vi "Configure Width Trigger Source [WT] Core.vi"(0 "IVI_Scope in":refnum<class "IVI_Scope.lvclass">, 1 "trigger source (\"CHANNEL1\")":string(combo)="CHANNEL1", 2 "trigger level (0.0 V)":dbl[unit] format="%.3f", 3 "width condition (Within)":i32(ring)=1 items=["Within"=1, "Outside"=2], 4 "width polarity (Positive)":i32(ring)=1 items=["Positive"=1, "Negative"=2], 5 "error in (no error)":errorcluster, 6 "width low threshold (1.0 E-9 V)":dbl[unit]=1e-09 format="%^.3e", 8 "width high threshold (2.0 E-9 V)":dbl[unit]=2e-09 format="%^.3e") -> (14 "IVI_Scope out":refnum<class "IVI_Scope.lvclass">, 19 "error out":errorcluster)   [LabVIEW 2013, in "IVI_Scope.lvlib" / "IVI_Scope.lvclass"]
doc: "This VI configures the width trigger. A width trigger occurs when the oscilloscope detects a positive or negative pulse with a width between, or optionally outside, the width thresholds. You specify the width thresholds with the Width Low Threshold and Width High Threshold parameters. You specify whether the oscilloscope triggers on pulse widths that are within or outside the width thresholds with the Width Condition parameter. You specify the polarity of the pulse with the Width Polarity parameter. The trigger does not actually occur until the edge of a pulse that corresponds to the Width Low Threshold, Width High Threshold, Width Condition, and Width Polarity crosses the threshold you specify in the Trigger Level parameter.\n\nNote (1) This VI affects instrument behavior only if the trigger type is IVISCOPE_VAL_WIDTH_TRIGGER. Call the IviScope Configure Trigger and IviScope Configure Trigger Coupling VIs to set the trigger type and trigger coupling before calling this VI.\n(2) This VI is part of the IviScopeWidthTrigger [WT] extension group."
uses:
  IVI_Scope.lvclass
  IVI_Scope.lvclass/IVI_Scope.ctl
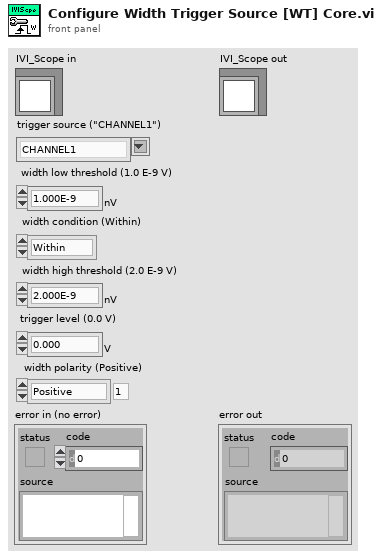
[diagram p1: front panel]
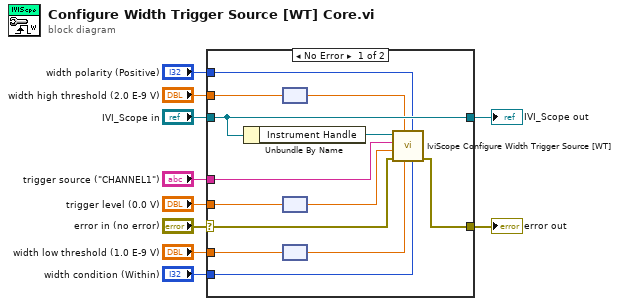
[diagram p0: block diagram]
diagram:
  n1 = case shown="No Error" "error in (no error)" {
    selector: "error in (no error)" -> [w21 w25]
    tunnel: [w20 w25] -> w9
    tunnel: [w23 w24] -> w7
    tunnel: "IVI_Scope in" -> [w23 w24]
    tunnel: "trigger source (\"CHANNEL1\")" -> [w19 _]
    tunnel: "trigger level (0.0 V)" -> [w18 _]
    tunnel: "width low threshold (1.0 E-9 V)" -> [w17 _]
    tunnel: "width condition (Within)" -> [w16 _]
    tunnel: "width high threshold (2.0 E-9 V)" -> [w14 _]
    tunnel: "width polarity (Positive)" -> [w15 _]
    frame No Error {
      n2 = Unbundle By Name(w23) -> ("Instrument Handle"=w22:refnum<k15>)
      n3 = node(w14) -> (w13:dbl)
      n4 = node(w18) -> (w12:dbl)
      n5 = node(w17) -> (w11:dbl)
      n6 = call <vilib>:"IviScope Configure Width Trigger Source [WT].vi"("width condition (Within)"=w16, "width polarity (Positive)"=w15, "width low threshold (1.0 E-9 V)"=w11, "width high threshold (2.0 E-9 V)"=w13, "error in (no error)"=w21, "trigger level (0.0 V)"=w12, "trigger source (\"CHANNEL1\")"=w19, "instrument handle"=w22) -> ("error out"=w20:errorcluster)  [unwired: 2 in, 1 out]
    }
    frame Error {
    }
  }
  "error out" <- w9
  "IVI_Scope out" <- w7
